vi "DefBallPosSkillVSS.vi"(8 "error in (no error)":errorcluster, 9 "Game":refnum<class "Game.lvclass">, 10 "Robot in":refnum<class "Robot.lvclass">, 11 "DefBallPosSkillVSS in":refnum<class "DefBallPosSkillVSS.lvclass">) -> (0 "error out":errorcluster, 2 "Robot out":refnum<class "Robot.lvclass">, 3 "DefBallPosSkillVSS out":refnum<class "DefBallPosSkillVSS.lvclass">)   [LabVIEW 2023, in "DefBallPosSkillVSS.lvclass"]
uses:
  DefBallPosSkillVSS.lvclass
  Robot_class/Robot.lvclass
  Game_class/Game.lvclass
  Object_class/Object.lvclass/Object.ctl
  Game_class/Game.lvclass/Game.ctl
  Robot_class/Robot.lvclass/Robot.ctl
  Game_class/Read EnemyRef.vi
  Game_class/Read BallRef.vi
  Game_class/Read FieldRef.vi
  Object_class/Read x.vi
  Object_class/Read y.vi
  Robot_class/Write dest_x.vi
  Robot_class/Write dest_y.vi
  Robot_class/Write dest_orientation.vi
  Ball_class/Ball.lvclass
  Enemy_class/Enemy.lvclass
  Field_class/Field.lvclass
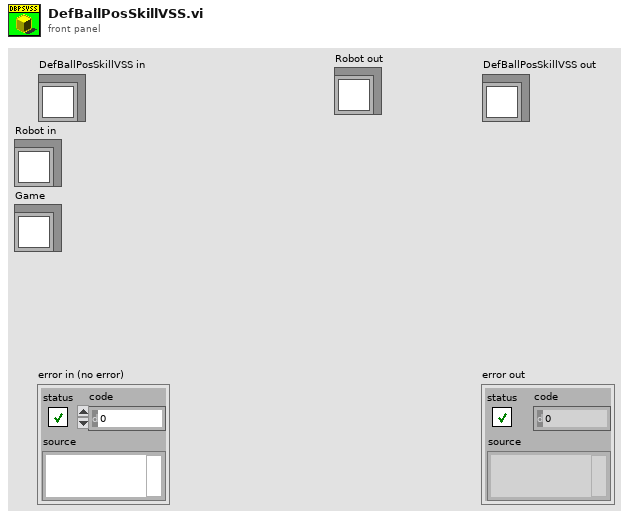
[diagram p1: front panel]
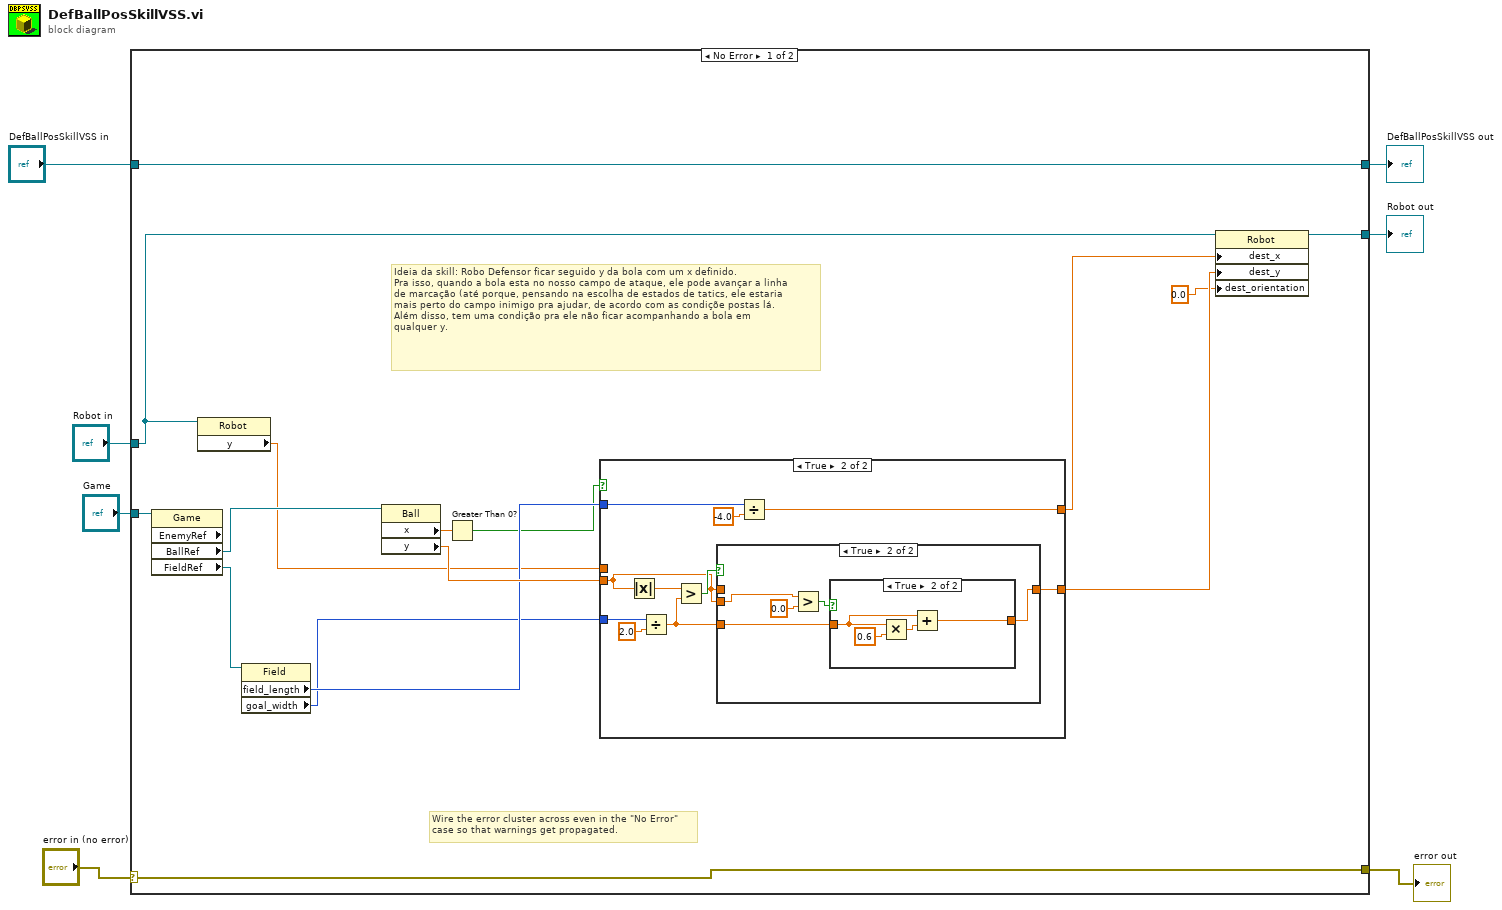
[diagram p0: block diagram]
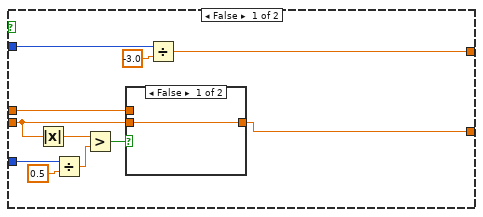
[diagram p2: hidden frame]
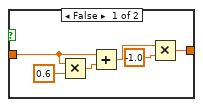
[diagram p5: hidden frame]
diagram:
  n1 = case shown="No Error" "error in (no error)" {
    selector: "error in (no error)" -> [w22 w65]
    tunnel: [w22 w65] -> w6
    tunnel: [w23 w64] -> w4
    tunnel: "DefBallPosSkillVSS in" -> [w23 w64]
    tunnel: "Robot in" -> [w12 w63]
    tunnel: [w21 w63] -> w2
    tunnel: "Game" -> [w20 _]
    frame No Error {
      # "Ideia da skill: Robo Defensor ficar seguido y da bola com um x definido.\nPra isso, quando a bola esta no nosso campo de ataque, ele pode avançar a linha\nde marcação (até porque, pensando na escolha de estados de tatics, ele estaria\nmais perto do campo inimigo pra ajudar, de acordo com as condiçõe postas lá.\nAlém disso, tem uma condição pra ele não ficar acompanhando a bola em\nqualquer y."
      # "Wire the error cluster across even in the \"No Error\"\ncase so that warnings get propagated."
      n2 = property class="Game" props=["EnemyRef", "BallRef", "FieldRef"](reference=w20) -> ("BallRef"=w19:refnum<class "Ball.lvclass">, "FieldRef"=w18:refnum<class "Field.lvclass">)  [unwired: 1 in, 3 out]
      n3 = property class="Robot"(reference=w12) -> ("y"=w11:dbl)  [unwired: 1 in, 2 out]
      n4 = property class="Field"(reference=w18) -> ("field_length"=w15:i32, "goal_width"=w13:i32)  [unwired: 1 in, 2 out]
      n5 = property class="Ball"(reference=w19) -> ("x"=w9:dbl, "y"=w16:dbl)  [unwired: 1 in, 2 out]
      n6 = Greater Than 0?(x=w9) -> (x > 0?=w8:bool)
      n7 = case shown="True" w8 {
        tunnel: [w25 w39] -> w17
        tunnel: w16 -> [w26 w37]
        tunnel: w15 -> [w33 w46]
        tunnel: [w32 w44] -> w14
        tunnel: w13 -> [w30 w40]
        tunnel: w11 -> [w24 _]
        frame False {
          n8 = Absolute Value(x=w26) -> (abs(x)=w31:dbl)
          n9 = Divide(x=w30, y=0.5) -> (x/y=w27:dbl)
          n10 = Greater?(x=w31, y=w27) -> (0:w28:bool)
          n11 = case shown="False" w28 {
            tunnel: w26 -> [w35 _]
            tunnel: [w35 w36] -> w25
            tunnel: w24 -> [_ w36]
            frame False {
            }
            frame True {
            }
          }
          n12 = Divide(x=w33, y=-3.0) -> (x/y=w32:dbl)
        }
        frame True {
          n13 = Absolute Value(x=w37) -> (abs(x)=w43:dbl)
          n14 = Divide(x=w40, y=2.0) -> (x/y=w38:dbl)
          n15 = Greater?(x=w43, y=w38) -> (0:w41:bool)
          n16 = case shown="True" w41 {
            tunnel: [w47 w48] -> w39
            tunnel: w37 -> [w47 _]
            tunnel: w38 -> [_ w49]
            tunnel: w37 -> [_ w52]
            frame False {
            }
            frame True {
              n17 = Greater?(x=w52, y=0.0) -> (0:w50:bool)
              n18 = case shown="True" w50 {
                tunnel: w49 -> [w53 w62]
                tunnel: [w54 w59] -> w48
                frame False {
                  n19 = Multiply(x=w53, y=0.6) -> (x*y=w57:dbl)
                  n20 = Add(x=w53, y=w57) -> (x+y=w56:dbl)
                  n21 = Multiply(x=w56, y=-1.0) -> (x*y=w54:dbl)
                }
                frame True {
                  n22 = Multiply(x=w62, y=0.6) -> (x*y=w60:dbl)
                  n23 = Add(x=w62, y=w60) -> (x+y=w59:dbl)
                }
              }
            }
          }
          n24 = Divide(x=w46, y=-4.0) -> (x/y=w44:dbl)
        }
      }
      n25 = property class="Robot"(reference=w12, "dest_x"=w14, "dest_y"=w17, "dest_orientation"=0.0) -> (reference out=w21:refnum<class "Robot.lvclass">)  [unwired: 1 in, 1 out]
    }
    frame Error {
    }
  }
  "error out" <- w6
  "DefBallPosSkillVSS out" <- w4
  "Robot out" <- w2
